vi "3rd_ac_Vir_humid_air_2024.vi"(8 "CO2 content (ppm)":dbl, 9 "Water Vapor Mole Fraction":dbl, 10 "Temperature [K]":dbl format="%.4g", 11 "Type of air":i32(listbox)=4) -> (2 "3rd ac press Virial [G]":dbl format="%.2g", 3 "3rd ac density Virial [L]":dbl format="%_6g", 4 "Lcw":dbl, 5 "Lbbw":dbl format="%#_6e", 6 "Lcd":dbl, 7 "Lbbd":dbl)   [LabVIEW 2016]
uses:
  2022/SOS_Global_2022.vi
panel:
  # "m^6 / mol^2"
  # "Pa^-2"
  # "m^3 / mol"
  # "m^3 / mol"
  # "m^6 / mol^2"
  # "m^6 / mol^2"
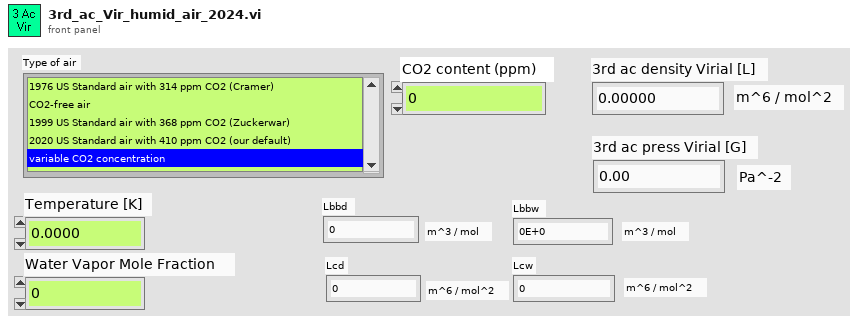
[diagram p1: front panel]
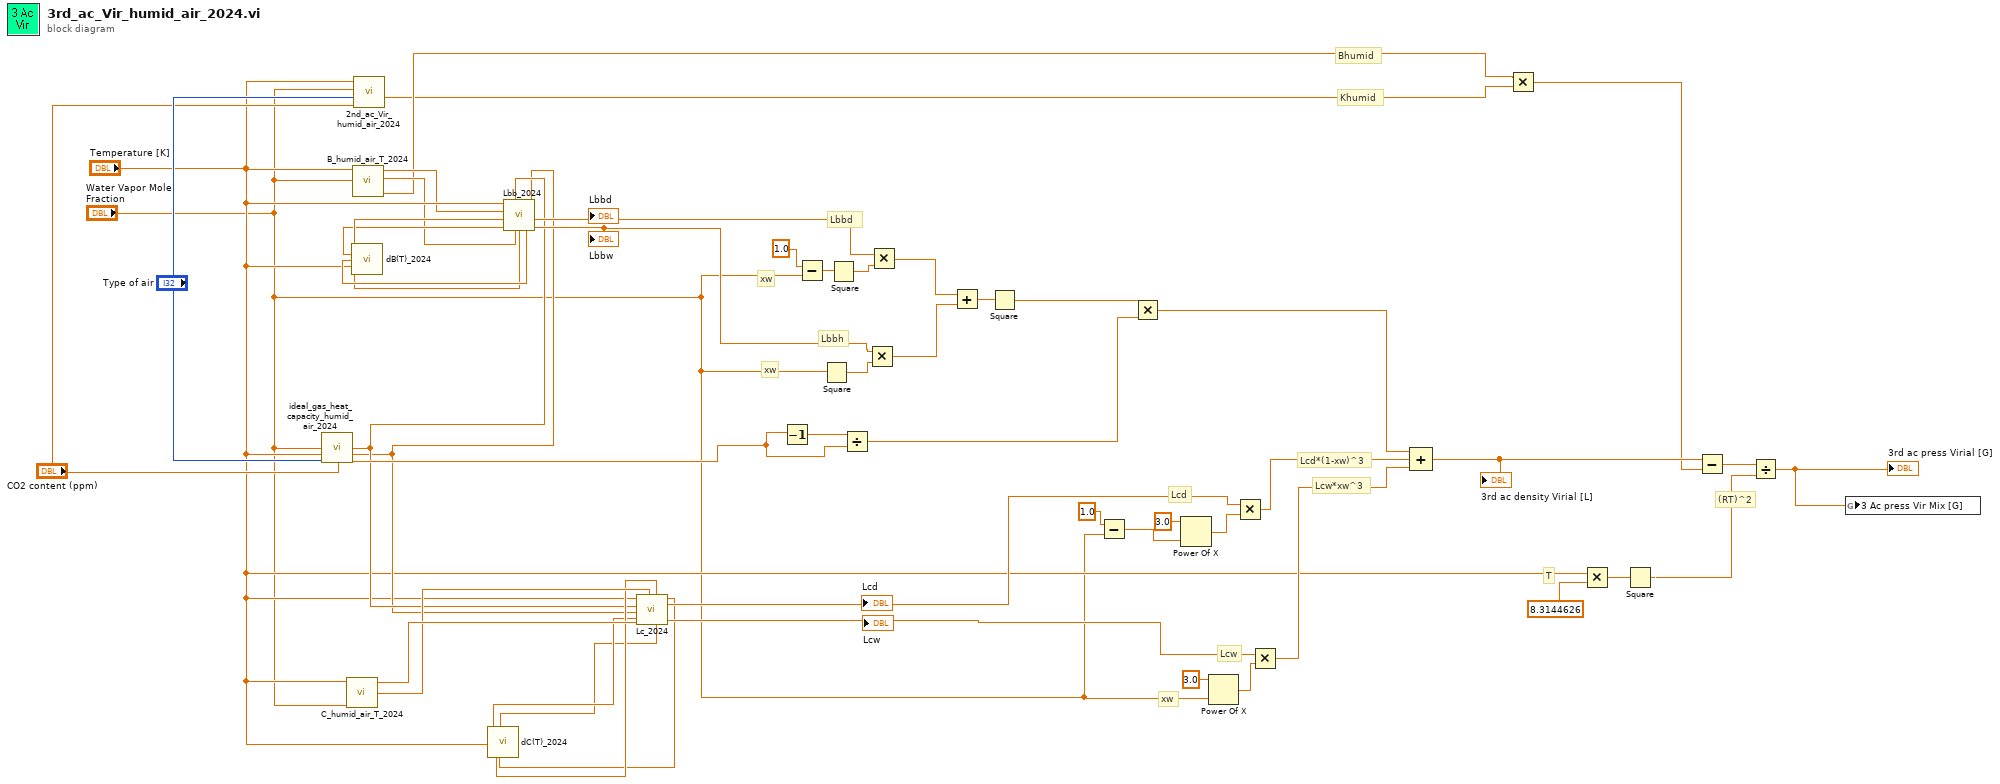
[diagram p0: block diagram]
diagram:
  # "Lcd*(1-xw)^3"
  # "Lcw*xw^3"
  # "Khumid"
  # "Bhumid"
  # "(RT)^2"
  # "T"
  # "xw"
  # "xw"
  # "xw"
  # "Lcw"
  # "Lcd"
  # "Lbbh"
  # "Lbbd"
  n1 = call "ideal_gas_heat_capacity_humid_air_2024.vi"("molar fraction of water vapor"="Water Vapor Mole Fraction", "Temperature [K]"="Temperature [K]", "Type of air"="Type of air", "CO2 content (ppm)"="CO2 content (ppm)") -> ("Gamma0 dry"=w14:dbl, "Gamma0 water"=w13:dbl, "Gamma0 humid air"=w15:dbl)  [unwired: 2 in, 7 out]
  n2 = call "C_humid_air_T_2024.vi"("xw molar fraction water vapor"="Water Vapor Mole Fraction", "Temperature (K)"="Temperature [K]") -> ("C water (m^3/mol)^2"=w22:dbl, "C dryair (m^3/mol)^2"=w23:dbl)  [unwired: 2 in, 1 out]
  n3 = call "dB(T)_2024.vi"("Temperature (K)"="Temperature [K]") -> ("dBair/dT"=w27:dbl, "d^2Bair/dT^2"=w26:dbl, "d^2Bwater/dT^2"=w25:dbl, "dBwater/dT"=w24:dbl)  [unwired: 3 in, 8 out]
  n4 = call "B_humid_air_T_2024.vi"("xw molar fraction water vapor"="Water Vapor Mole Fraction", "Temperature (K)"="Temperature [K]") -> ("Bhumid air (xw,T) [m^3/mol]"=w2:dbl, "Bw(T) [m^3/mol]"=w6:dbl, "Bd(T) [m^3/mol]"=w7:dbl)  [unwired: 5 in, 2 out]
  n5 = call "2nd_ac_Vir_humid_air_2024.vi"("CO2 content (ppm)"="CO2 content (ppm)", "Type of air"="Type of air", "xw molar fraction water vapor"="Water Vapor Mole Fraction", "Temperature (K)"="Temperature [K]") -> ("2nd ac vir humid air \"K\""=w1:dbl)  [unwired: 3 out]
  n6 = call "dC(T)_2024.vi"("Temperature (K)"="Temperature [K]") -> ("dCa/dT"=w19:dbl, "d^2Ca/dT^2"=w18:dbl, "dCw/dT"=w21:dbl, "d^2Cw/dT^2"=w20:dbl)  [unwired: 1 in, 4 out]
  n7 = call "Lbb_2024.vi"("Gamma_w"=w13, "d^2Bw(T)/dT^2"=w25, "dBw(T)/dT"=w24, "Bw(T)"=w6, "Gamma_dryair"=w14, "d^2Bd(T)/dT^2"=w26, "dBd(T)/dT"=w27, "Bd(T)"=w7, "Temperature [K]"="Temperature [K]") -> ("Lbbw"=w32:dbl, "Lbbd"=w33:dbl)  [unwired: 1 in]
  "Lbbd" <- w33
  "Lbbw" <- w32
  n8 = call "Lc_2024.vi"("d^2Cw(T)/dT^2"=w20, "d^2Cd(T)/dT^2"=w18, "dCw(T)/dT"=w21, "dCd(T)/dT"=w19, "Cw(T)"=w22, "Cd(T)"=w23, "Gamma0_water"=w13, "Gamma0_dry air"=w14, "Temperature [K]"="Temperature [K]") -> ("Lcw"=w30:dbl, "Lcd"=w31:dbl)  [unwired: 1 in]
  "Lcd" <- w31
  "Lcw" <- w30
  n9 = Decrement(x=w15) -> (x-1=w17:dbl)
  n10 = Subtract(x=1.0, y="Water Vapor Mole Fraction") -> (x-y=w34:dbl)
  n11 = Square(x="Water Vapor Mole Fraction") -> (x^2=w38:dbl)
  n12 = Square(x=w34) -> (x^2=w35:dbl)
  n13 = Divide(x=w17, y=w15) -> (x/y=w42:dbl)
  n14 = Multiply(x=w32, y=w38) -> (x*y=w39:dbl)
  n15 = Multiply(x=w33, y=w35) -> (x*y=w37:dbl)
  n16 = Add(x=w37, y=w39) -> (x+y=w40:dbl)
  n17 = Square(x=w40) -> (x^2=w41:dbl)
  n18 = Subtract(x=1.0, y="Water Vapor Mole Fraction") -> (x-y=w3:dbl)
  n19 = Multiply(x=w41, y=w42) -> (x*y=w47:dbl)
  n20 = Power Of X(1:w3, 2:3.0 ("y")) -> (0:w44:dbl)
  n21 = Power Of X(1:"Water Vapor Mole Fraction", 2:3.0 ("y")) -> (0:w46:dbl)
  n22 = Multiply(x=w31, y=w44) -> (x*y=w48:dbl)
  n23 = Multiply(x=w30, y=w46) -> (x*y=w49:dbl)
  n24 = Compound Arithmetic op=ADD(w47, w48, w49) -> (w16:dbl)
  "3rd ac density Virial [L]" <- w16
  n25 = Multiply(x=w2, y=w1) -> (x*y=w11:dbl)
  n26 = Multiply(x="Temperature [K]", y=8.3144626) -> (x*y=w51:dbl)
  n27 = Square(x=w51) -> (x^2=w28:dbl)
  n28 = Subtract(x=w16, y=w11) -> (x-y=w29:dbl)
  n29 = Divide(x=w29, y=w28) -> (x/y=w12:dbl)
  "3rd ac press Virial [G]" <- w12
  n30 = global write "SOS_Global_2022.vi" "3 Ac press Vir Mix [G]"(w12) -> ()
